vi "subXMLFindNodeValueFromName.vi"(9 "Property value":string, 10 "Property name":string, 11 "Refnum in":refnum<k20>) -> (1 "Value":string, 2 "Found?":bool, 3 "Refnum out":refnum<k20>)   [LabVIEW 2020, in "SolutionBuilder.lvlib"]
uses:
  SolutionBuilder.lvlib
  <resource>/objmgr/DOMUserDefRef.rc
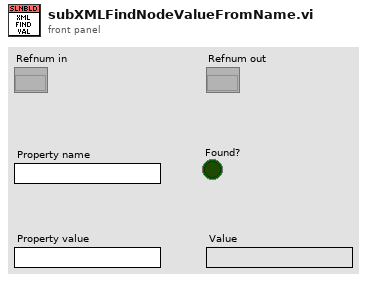
[diagram p1: front panel]
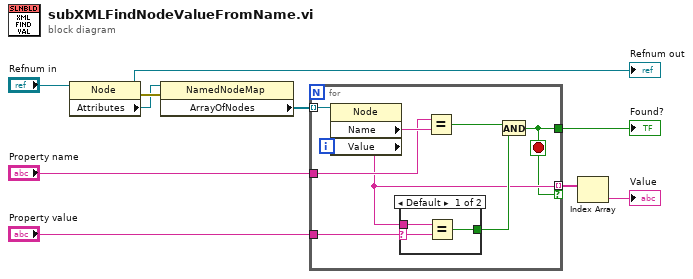
[diagram p0: block diagram]
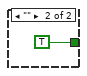
[diagram p2: hidden frame]
diagram:
  n1 = property class="Node"(reference="Refnum in") -> (reference out=→"Refnum out":refnum<k20>, error out=w3:errorcluster, "Attributes"=w1:refnum<k20>)  [unwired: 1 in]
  n2 = property class="NamedNodeMap"(reference=w1, error in=w3) -> ("ArrayOfNodes"=w2:refnum<k20>[])  [unwired: 2 out]
  n3 = for {
    tunnel: w2 -> [w18] mode=indexing
    tunnel: [w12] -> w8
    tunnel: "Property name" -> [w14]
    tunnel: "Property value" -> [w11]
    tunnel: [w13] -> w9 mode=indexing if=w12
    stop <- w12 stop-if-true
    n4 = property class="Node"(reference=w18) -> ("Name"=w17:string, "Value"=w13:string)  [unwired: 1 in, 2 out]
    n5 = case shown="Default" w11 {
      selector: w11 -> [w19 _]
      tunnel: [w21 TRUE] -> w15
      tunnel: w13 -> [w20 _]
      frame Default {
        n6 = Equal?(x=w20, y=w19) -> (x = y?=w21:bool)
      }
      frame "" {
      }
    }
    n7 = Equal?(x=w14, y=w17) -> (x = y?=w16:bool)
    n8 = And(x=w16, y=w15) -> (x .and. y?=w12:bool)
  }
  "Found?" <- w8
  n9 = Index Array(array=w9) -> (element=→"Value":string)  [unwired: 1 in]
